vi "Close Log.vi"(8 "error in":errorcluster) -> (0 "error out":errorcluster)   [LabVIEW 2015, in "Generic Module Library.lvlib" / "Template G_Module.lvlib"]
uses:
  Template G_Module.lvlib
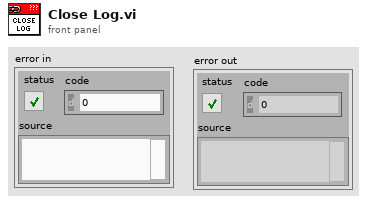
[diagram p1: front panel]
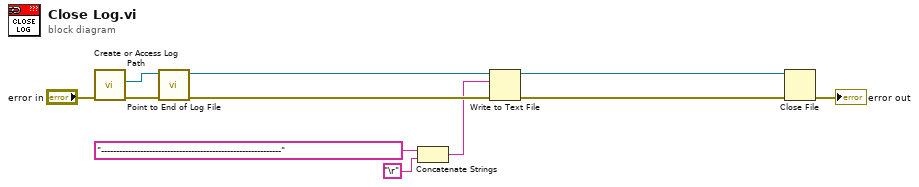
[diagram p0: block diagram]
diagram:
  n1 = call "Create or Access Log Path.vi"("error in"="error in") -> ("error out"=w9:errorcluster, "Log Refnum Out"=w7:refnum<file>)  [unwired: 7 in, 2 out]
  n2 = call "Point to End of Log File.vi"("error in (no error)"=w9, "Byte Stream File in"=w7) -> ("error out"=w8:errorcluster, "Byte Stream File out"=w5:refnum<file>)  [unwired: 8 in]
  n3 = Concatenate Strings("------------------------------------------------------------" ("text"), "\r") -> (w2:string)
  n4 = Write to Text File(file (use dialog)=w5, text=w2, error in=w8) -> (refnum out=w4:refnum<file>, error out=w6:errorcluster)  [unwired: 1 in, 1 out]
  n5 = Close File(refnum=w4, error in=w6) -> (error out=→"error out":errorcluster)  [unwired: 1 out]
